vi "RichToFlatcif_manager_QueryPluginInfoResponse.vi"(5 "OutputClusterType":T1, 11 "InputCluster":T16) -> (3 "OutputCluster":T1)   [LabVIEW 2021, in "CIF_Manager_client.lvlib"]
uses:
  cif_manager_QueryPluginInfoResponse.ctl
  cif_manager_PluginInfoArray.ctl
  cif_manager_PluginInfo.ctl
  cif_common_ShortVersion.ctl
  cif_management_common_PluginStatusData.ctl
  cif_management_common_PluginStatusData_PluginState.ctl
  cif_management_common_TimingStatistics.ctl
  cif_common_TimingStats.ctl
  cif_management_common_FifoStatistics.ctl
  cif_management_common_Error.ctl
  cif_management_common_MonitorDoubles.ctl
  cif_management_common_MonitorU64.ctl
  cif_management_common_MonitorI64.ctl
  cif_management_common_LoaderInfo.ctl
  cif_management_common_LoaderType.ctl
  cif_manager_QueryPluginInfoResponse_Flat.ctl
  cif_manager_PluginInfoArray_Flat.ctl
  cif_manager_PluginInfo_Flat.ctl
  cif_common_ShortVersion_Flat.ctl
  cif_management_common_PluginStatusData_Flat.ctl
  cif_management_common_TimingStatistics_Flat.ctl
  cif_common_TimingStats_Flat.ctl
  cif_management_common_FifoStatistics_Flat.ctl
  cif_management_common_Error_Flat.ctl
  cif_management_common_MonitorDoubles_Flat.ctl
  cif_management_common_MonitorU64_Flat.ctl
  cif_management_common_MonitorI64_Flat.ctl
  cif_management_common_LoaderInfo_Flat.ctl
  CIF_Manager_client.lvlib
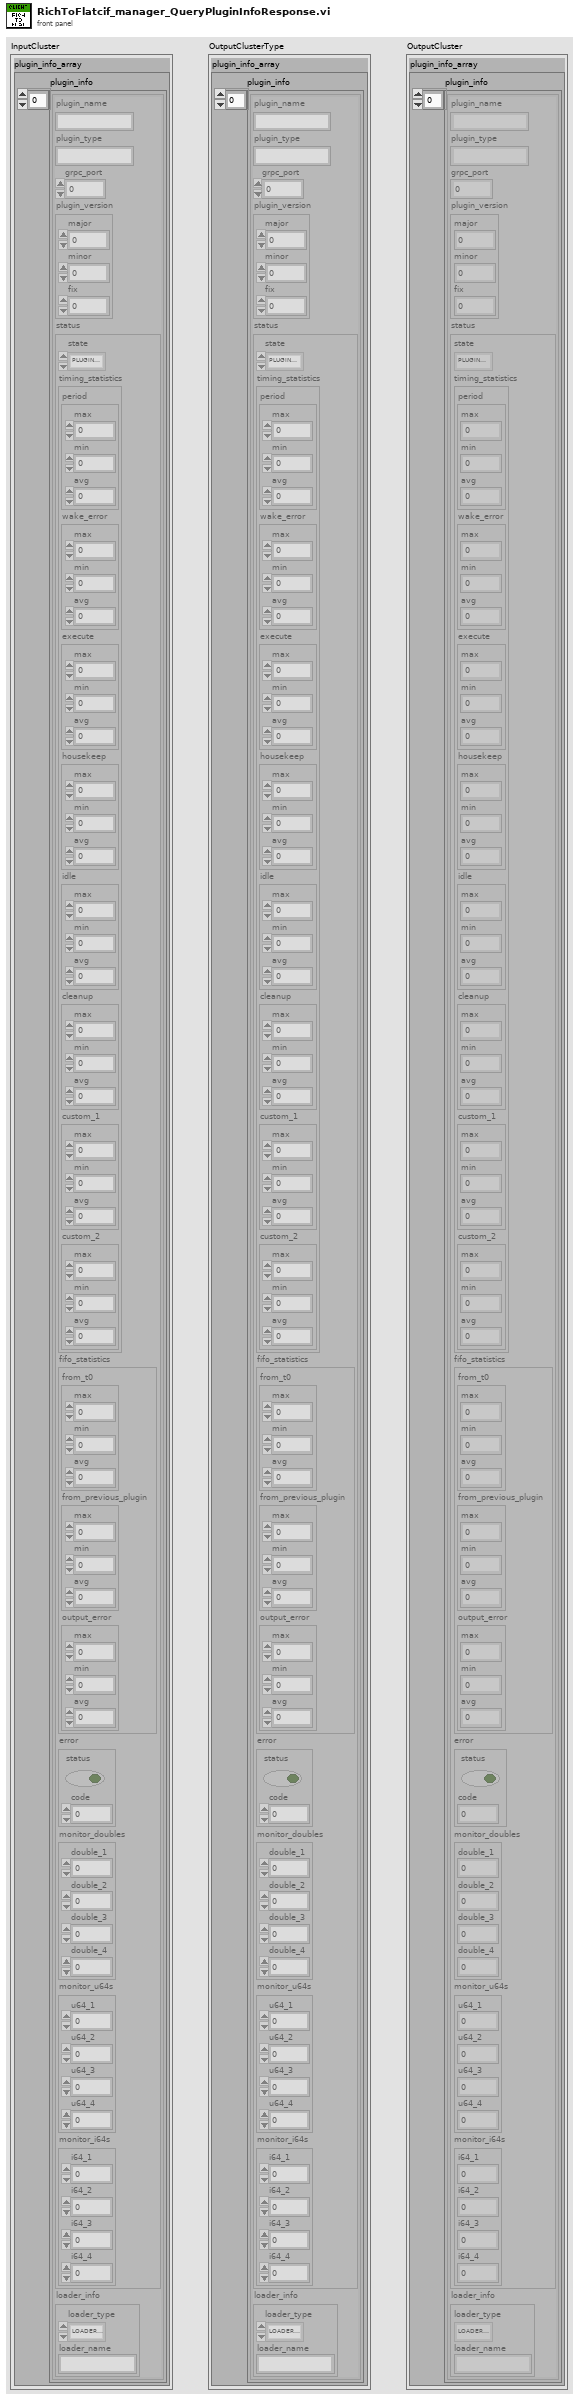
[diagram p1: front panel]
types:
  T1 = typedef "CIF_Manager_client.lvlib/cif_manager_QueryPluginInfoResponse_Flat.ctl" = cluster{"plugin_info_array":T2}
  T2 = typedef "CIF_Manager_client.lvlib/cif_manager_PluginInfoArray_Flat.ctl" = cluster{"plugin_info":T3[]}
  T3 = typedef "CIF_Manager_client.lvlib/cif_manager_PluginInfo_Flat.ctl" = cluster{"plugin_name":string, "plugin_type":string, "grpc_port":i32, "plugin_version":T4, "status":T5, "loader_info":T14}
  T4 = typedef "CIF_Manager_client.lvlib/cif_common_ShortVersion_Flat.ctl" = cluster{"major":u32, "minor":u32, "fix":u32}
  T5 = typedef "CIF_Manager_client.lvlib/cif_management_common_PluginStatusData_Flat.ctl" = cluster{"state":T6, "timing_statistics":T7, "fifo_statistics":T9, "error":T10, "monitor_doubles":T11, "monitor_u64s":T12, "monitor_i64s":T13}
  T6 = typedef "CIF_Manager_client.lvlib/cif_management_common_PluginStatusData_PluginState.ctl" = enum32{"PLUGINSTATE_UNKNOWN", "PLUGINSTATE_CREATING", "PLUGINSTATE_LISTENING", "PLUGINSTATE_RUNNING", "PLUGINSTATE_CLEANINGUP", "PLUGINSTATE_DESTROYING", "PLUGINSTATE_PREPARED", "PLUGINSTATE_FTE_RUN"}
  T7 = typedef "CIF_Manager_client.lvlib/cif_management_common_TimingStatistics_Flat.ctl" = cluster{"period":T8, "wake_error":T8, "execute":T8, "housekeep":T8, "idle":T8, "cleanup":T8, "custom_1":T8, "custom_2":T8}
  T8 = typedef "CIF_Manager_client.lvlib/cif_common_TimingStats_Flat.ctl" = cluster{"max":i64, "min":i64, "avg":dbl}
  T9 = typedef "CIF_Manager_client.lvlib/cif_management_common_FifoStatistics_Flat.ctl" = cluster{"from_t0":T8, "from_previous_plugin":T8, "output_error":T8}
  T10 = typedef "CIF_Manager_client.lvlib/cif_management_common_Error_Flat.ctl" = cluster{"status":bool, "code":i32}
  T11 = typedef "CIF_Manager_client.lvlib/cif_management_common_MonitorDoubles_Flat.ctl" = cluster{"double_1":dbl, "double_2":dbl, "double_3":dbl, "double_4":dbl}
  T12 = typedef "CIF_Manager_client.lvlib/cif_management_common_MonitorU64_Flat.ctl" = cluster{"u64_1":u64, "u64_2":u64, "u64_3":u64, "u64_4":u64}
  T13 = typedef "CIF_Manager_client.lvlib/cif_management_common_MonitorI64_Flat.ctl" = cluster{"i64_1":i64, "i64_2":i64, "i64_3":i64, "i64_4":i64}
  T14 = typedef "CIF_Manager_client.lvlib/cif_management_common_LoaderInfo_Flat.ctl" = cluster{"loader_type":T15, "loader_name":string}
  T15 = typedef "CIF_Manager_client.lvlib/cif_management_common_LoaderType.ctl" = enum32{"LOADERTYPE_UNKNOWN", "LOADERTYPE_LABVIEW"}
  T16 = typedef "CIF_Manager_client.lvlib/cif_manager_QueryPluginInfoResponse.ctl" = cluster{"plugin_info_array":T17}
  T17 = typedef "CIF_Manager_client.lvlib/cif_manager_PluginInfoArray.ctl" = cluster{"plugin_info":T18[]}
  T18 = typedef "CIF_Manager_client.lvlib/cif_manager_PluginInfo.ctl" = cluster{"plugin_name":string, "plugin_type":string, "grpc_port":i32, "plugin_version":T19, "status":T20, "loader_info":T28}
  T19 = typedef "CIF_Manager_client.lvlib/cif_common_ShortVersion.ctl" = cluster{"major":u32, "minor":u32, "fix":u32}
  T20 = typedef "CIF_Manager_client.lvlib/cif_management_common_PluginStatusData.ctl" = cluster{"state":T6, "timing_statistics":T21, "fifo_statistics":T23, "error":T24, "monitor_doubles":T25, "monitor_u64s":T26, "monitor_i64s":T27}
  T21 = typedef "CIF_Manager_client.lvlib/cif_management_common_TimingStatistics.ctl" = cluster{"period":T22, "wake_error":T22, "execute":T22, "housekeep":T22, "idle":T22, "cleanup":T22, "custom_1":T22, "custom_2":T22}
  T22 = typedef "CIF_Manager_client.lvlib/cif_common_TimingStats.ctl" = cluster{"max":i64, "min":i64, "avg":dbl}
  T23 = typedef "CIF_Manager_client.lvlib/cif_management_common_FifoStatistics.ctl" = cluster{"from_t0":T22, "from_previous_plugin":T22, "output_error":T22}
  T24 = typedef "CIF_Manager_client.lvlib/cif_management_common_Error.ctl" = cluster{"status":bool, "code":i32}
  T25 = typedef "CIF_Manager_client.lvlib/cif_management_common_MonitorDoubles.ctl" = cluster{"double_1":dbl, "double_2":dbl, "double_3":dbl, "double_4":dbl}
  T26 = typedef "CIF_Manager_client.lvlib/cif_management_common_MonitorU64.ctl" = cluster{"u64_1":u64, "u64_2":u64, "u64_3":u64, "u64_4":u64}
  T27 = typedef "CIF_Manager_client.lvlib/cif_management_common_MonitorI64.ctl" = cluster{"i64_1":i64, "i64_2":i64, "i64_3":i64, "i64_4":i64}
  T28 = typedef "CIF_Manager_client.lvlib/cif_management_common_LoaderInfo.ctl" = cluster{"loader_type":T15, "loader_name":string}
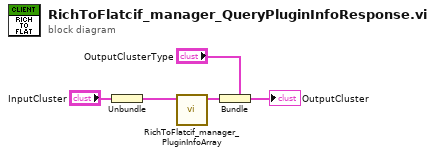
[diagram p0: block diagram]
diagram:
  n1 = Unbundle "Unbundle"("InputCluster") -> ("plugin_info_array"=w2:T17)
  n2 = call "RichToFlatcif_manager_PluginInfoArray.vi"("InputCluster"=w2) -> ("OutputCluster"=w1:T2)  [unwired: 10 in]
  n3 = Bundle "Bundle"(cluster="OutputClusterType", "plugin_info_array"=w1) -> (→"OutputCluster":T1)
